vi "按比例截取数组.vi"(10 "长度":dbl, 11 "X":dbl[](array[numeric])) -> (3 "Y":dbl[](array[numeric]))   [LabVIEW 2020]
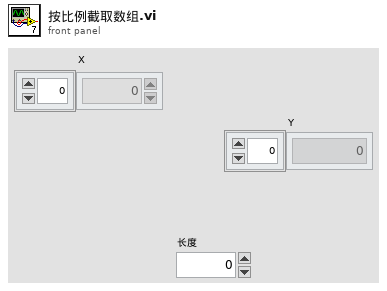
[diagram p1: front panel]
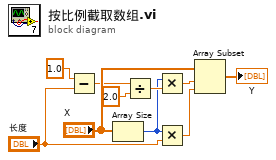
[diagram p0: block diagram]
diagram:
  n1 = Subtract(x=1.0, y="长度") -> (x-y=w8:dbl)
  n2 = Array Size(array="X") -> (size(s)=w3:i32)
  n3 = Divide(x=w8, y=2.0) -> (x/y=w6:dbl)
  n4 = Multiply(x=w3, y=w6) -> (x*y=w5:dbl)
  n5 = Multiply(x=w3, y="长度") -> (x*y=w2:dbl)
  n6 = Array Subset(array="X", index=w5, length=w2) -> (→"Y":dbl[])
